vi "configure runtime data.vi"(4 "output dictionary":refnum<class "data dictionary.lvclass">, 6 "input dictionary":refnum<class "data dictionary.lvclass">, 8 "error in":errorcluster, 10 "Slave Info List":T6(array[cluster]), 11 "Profibus Module configuration in":refnum<class "Profibus Module configuration.lvclass">) -> (0 "error out":errorcluster, 1 "diagnostics":T1[](array[typedef]), 2 "inputs":T3[](array[typedef]), 3 "outputs":T3[](array[typedef]), 5 "full command list":u32[](array[numeric]))   [LabVIEW 2013, in "Profibus Module runtime.lvclass"]
uses:
  Profibus Module runtime.lvclass
  configuration/Profibus Module configuration.lvclass
  profibus slave configuration.ctl
  profibus mapping configuration.ctl
  <vilib>/NI/Tag Bus/tag/Data Type.ctl
  <vilib>/NI/Tag Bus/dictionary/data dictionary.lvclass
  profibus diagnostics reporting.ctl
  configuration/error throw specification.ctl
  configuration/Profibus Module configuration.lvclass/Profibus Module configuration.ctl
  dynamic profibus/profibus master action.ctl
  <vilib>/NI/Tag Bus/tag/tag descriptor.lvclass/tag descriptor.ctl
  <vilib>/NI/Tag Bus/dictionary/data dictionary.lvclass/data dictionary.ctl
  configuration/Read slave diagnostics.vi
  <vilib>/NI/Tag Bus/dictionary/look up tag by type.vi
  <vilib>/NI/Tag Bus/dictionary/lookup polymorphs/locate Array of U8.vi
  <vilib>/NI/Tag Bus/tag/read tag name.vi
  <vilib>/NI/Tag Bus/dictionary/search/find data index.vi
  <vilib>/NI/Tag Bus/dictionary/search/search string list.vi
  <vilib>/NI/Tag Bus/dictionary/tag not found.vi
  dynamic profibus/dynamic profibus.lvlib
  <vilib>/NI/Tag Bus/tag/tag descriptor.lvclass
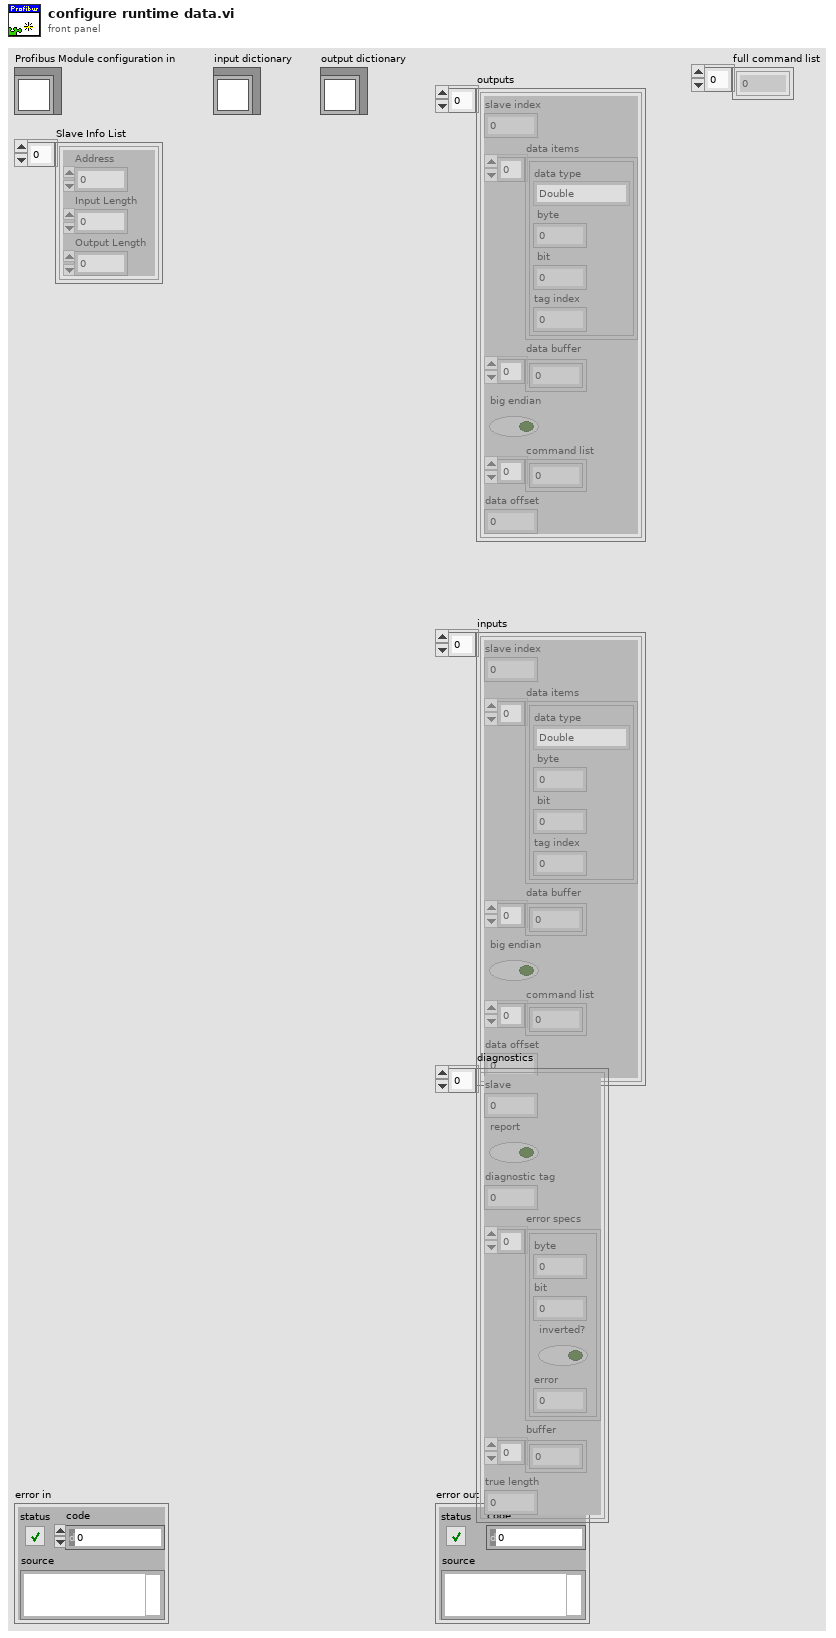
[diagram p1: front panel]
types:
  T1 = typedef "Profibus Module runtime.lvclass/profibus diagnostics reporting.ctl" = cluster{"slave":i8, "report":bool, "diagnostic tag":i32, "error specs":T2[], "buffer":u8[], "true length":u8}
  T2 = typedef "Profibus Module configuration.lvclass/error throw specification.ctl" = cluster{"byte":i32, "bit":i32, "inverted?":bool, "error":i32}
  T3 = typedef "Profibus Module runtime.lvclass/profibus slave configuration.ctl" = cluster{"slave index":i8, "data items":T4[], "data buffer":u8[], "big endian":bool, "command list":u32[], "data offset":u8}
  T4 = typedef "Profibus Module runtime.lvclass/profibus mapping configuration.ctl" = cluster{"data type":T5, " byte":i32, " bit":i32, "tag index":i32}
  T5 = typedef "tag bus.lvlib/tag descriptor.lvclass/Data Type.ctl" = enum16{"Double", "Single", "I64", "I32", "I16", "I8", "U64", "U32", "U16", "U8", "Boolean", "String", "Array of Double", "Array of Single", "Array of I64", "Array of I32", "Array of I16", "Array of I8", "Array of U64", "Array of U32", "Array of U16", "Array of U8", "Array of Boolean", "Array of String"}
  T6 = cluster{"Address":i8, "Input Length":u8, "Output Length":u8}[]
  T7 = typedef "Profibus Module configuration.lvclass/endianness setting.ctl" = cluster{"slave":i8, "big endian":bool}
  T8 = typedef "Profibus Module runtime.lvclass/required data sets.ctl" = cluster{"Address":i8, "Input Start":u8, "Input End":u8, "Output Start":u8, "Output End":u8, "chan in":refnum<class "Profibus channel.lvclass">[], "chan out":refnum<class "Profibus channel.lvclass">[]}
  T9 = typedef "dynamic profibus.lvlib/profibus master action.ctl" = enum8{"initialize", "uninitialize", "stop", "get input", "get input size", "set output", "get output size", "get diagnostic", "transfer data", "transfer diagnostics", "read many inputs"}
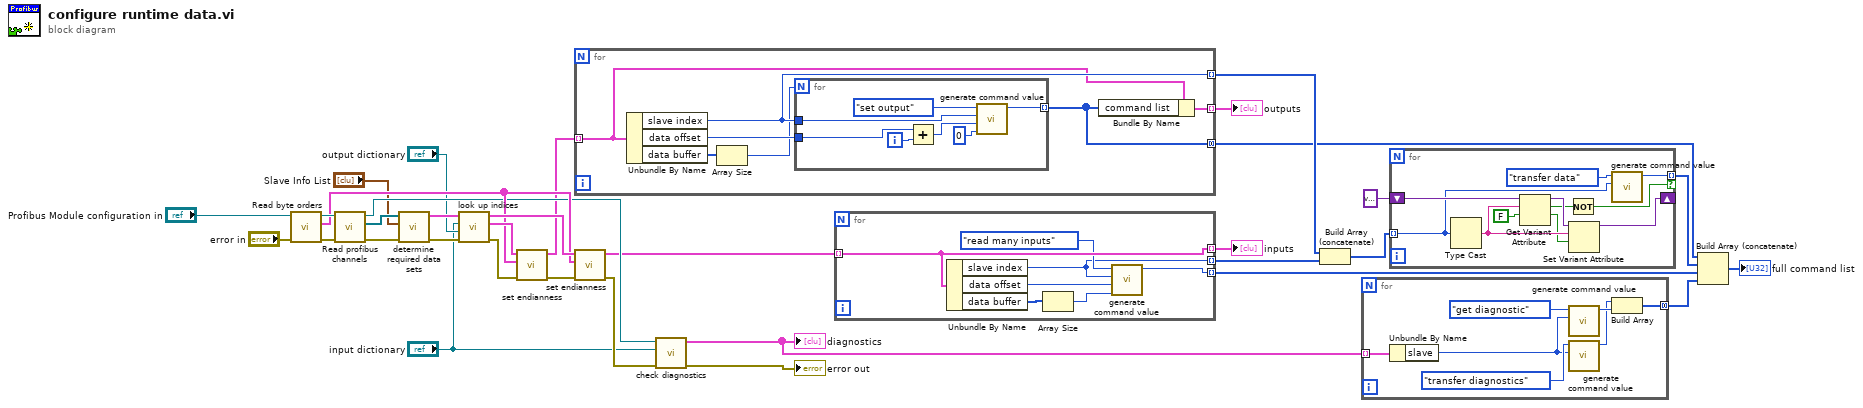
[diagram p0: block diagram]
diagram:
  n1 = call "Read byte orders.vi"("error in"="error in", "Profibus Module configuration in"="Profibus Module configuration in") -> ("error out"=w29:errorcluster, "byte orders"=w26:T7[], "Profibus Module configuration out"=w30:refnum<class "Profibus Module configuration.lvclass">)  [unwired: 7 in]
  n2 = call "Read profibus channels.vi"("error in"=w29, "Profibus Module configuration in"=w30) -> ("error out"=w11:errorcluster, "channels"=w10:refnum<class "Profibus channel.lvclass">[], "Profibus Module configuration out"=w23:refnum<class "Profibus Module configuration.lvclass">)  [unwired: 7 in]
  n3 = call "determine required data sets.vi"("error in"=w11, "Slave Info List"="Slave Info List", "channels"=w10) -> ("error out"=w7:errorcluster, "slave data subsets"=w6:T8[])  [unwired: 7 in]
  n4 = call "look up indices.vi"("error in"=w7, "output dictionary"="output dictionary", "input dictionary"="input dictionary", "slave data subsets"=w6) -> ("error out"=w8:errorcluster, "outputs"=w32:T3[], "inputs"=w33:T3[])  [unwired: 5 in]
  n5 = call "set endianness.vi"("error in"=w8, "byte orders"=w26, "config in"=w32) -> ("error out"=w27:errorcluster, "config out"=w20:T3[])  [unwired: 7 in]
  n6 = for {
    tunnel: w20 -> [w39] mode=indexing
    tunnel: [w38] -> w16 mode=concatenating
    tunnel: [w40] -> w18 mode=indexing
    tunnel: [w37] -> w14 mode=indexing
    n7 = Unbundle By Name(w39) -> ("slave index"=w40:i8, "data offset"=w36:u8, "data buffer"=w35:u8[])
    n8 = Array Size(array=w35) -> (size(s)=w34:i32)
    n9 = for {
      N: w34 -> [_]
      tunnel: [w47] -> w38 mode=indexing
      tunnel: w40 -> [w45]
      tunnel: w36 -> [w41]
      i -> [w44]
      n10 = Add(x=w41, y=w44) -> (x+y=w42:i32)
      n11 = call "generate command value.vi"("data"=u8 0, "index"=w42, "device"=w45, "action"=profibus_master_action."set output") -> ("Element"=w47:u32)  [unwired: 7 in]
    }
    n12 = Bundle By Name(cluster=w39, "command list"=w38) -> (w37:T3)
  }
  "outputs" <- w14
  n13 = call "set endianness.vi"("error in"=w27, "byte orders"=w26, "config in"=w33) -> ("error out"=w24:errorcluster, "config out"=w21:T3[])  [unwired: 7 in]
  n14 = call "check diagnostics.vi"("error in"=w24, "data dictionary in"="input dictionary", "Profibus Module configuration in"=w23) -> ("error out"=→"error out":errorcluster, "diagnostics"=w22:T1[])  [unwired: 7 in]
  "diagnostics" <- w22
  n15 = for {
    tunnel: w21 -> [w54] mode=indexing
    tunnel: [w53] -> w17 mode=indexing
    tunnel: [w51] -> w19 mode=indexing
    tunnel: [w54] -> w13 mode=indexing
    n16 = Unbundle By Name(w54) -> ("slave index"=w51:i8, "data offset"=w50:u8, "data buffer"=w49:u8[])
    n17 = Array Size(array=w49) -> (size(s)=w48:i32)
    n18 = call "generate command value.vi"("data"=w48, "index"=w50, "device"=w51, "action"=profibus_master_action."read many inputs") -> ("Element"=w53:u32)  [unwired: 7 in]
  }
  "inputs" <- w13
  n19 = Build Array (concatenate)(w18, w19) -> (w15:i8[])
  n20 = for {
    tunnel: w22 -> [w61] mode=indexing
    tunnel: [w58] -> w2 mode=concatenating
    n21 = Unbundle By Name(w61) -> ("slave"=w55:i8)
    n22 = call "generate command value.vi"("device"=w55, "action"=profibus_master_action."get diagnostic") -> ("Element"=w60:u32)  [unwired: 9 in]
    n23 = call "generate command value.vi"("device"=w55, "action"=profibus_master_action."transfer diagnostics") -> ("Element"=w59:u32)  [unwired: 9 in]
    n24 = Build Array(w59, w60) -> (w58:u32[])
  }
  n25 = for {
    tunnel: [w64] -> w3 mode=indexing if=w66
    tunnel: w15 -> [w62] mode=indexing
    shift-right: [w72] -> _
    shift-left: variant -> [w71]
    n26 = Type Cast(x=w62) -> (*(type *) &x=w69:string)  [unwired: 1 in]
    n27 = Get Variant Attribute(Variant=w71, name=w69, default value (empty Variant)=FALSE) -> (duplicate Variant=w70:variant, found=w67:bool, value=w65:bool)  [unwired: 1 in, 1 out]
    n28 = Not(x=w67) -> (.not. x?=w66:bool)
    n29 = Set Variant Attribute(Variant=w70, name=w69, value=w65) -> (Variant out=w72:variant)  [unwired: 1 in, 2 out]
    n30 = call "generate command value.vi"("device"=w62, "action"=profibus_master_action."transfer data") -> ("Element"=w64:u32)  [unwired: 9 in]
  }
  n31 = Build Array (concatenate)(w16, w3, w17, w2) -> (→"full command list":u32[])
